vi "transformedStadisticColumnInformation.vi"(8 "error in":errorcluster, 11 "columnInformationReading":T2(array[cluster])) -> (0 "error out":errorcluster, 3 "columnInformationReadingTransformed":string[](array[string]))   [LabVIEW 2014]
uses:
  <vilib>/addons/database/Auxilliary.llb/DB Tools DataTypes.ctl
  <vilib>/addons/database/NI_Database_API.lvlib
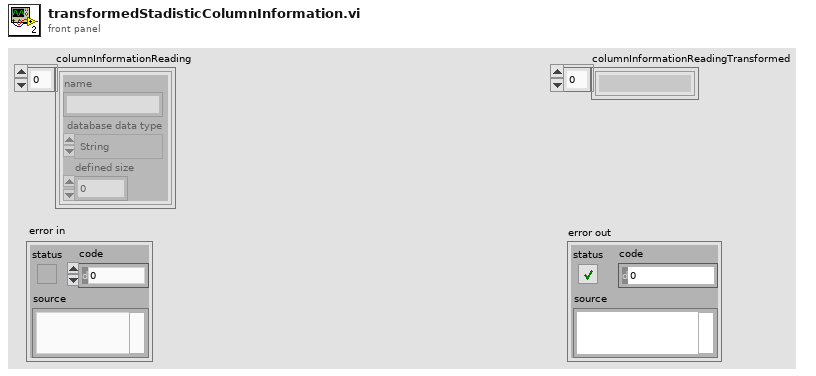
[diagram p1: front panel]
types:
  T1 = typedef "NI_Database_API.lvlib/DB Tools DataTypes.ctl" = enum16{"String", "Long (I32)", "Single (SGL)", "Double (DBL)", "Date/Time", "Binary"}
  T2 = cluster{"name":string, "database data type":T1, "defined size":i32}[]
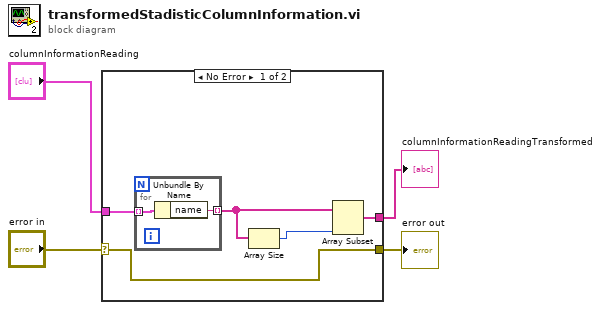
[diagram p0: block diagram]
diagram:
  n1 = case shown="No Error" "error in" {
    selector: "error in" -> [w6 w12]
    tunnel: "columnInformationReading" -> [w9 _]
    tunnel: [w8 _] -> w3
    tunnel: [w6 w12] -> w1
    frame No Error {
      n2 = for {
        tunnel: w9 -> [w10] mode=indexing
        tunnel: [w11] -> w7 mode=indexing
        n3 = Unbundle By Name(w10) -> ("name"=w11:string)
      }
      n4 = Array Size(array=w7) -> (size(s)=w5:i32)
      n5 = Array Subset(array=w7, length=w5) -> (w8:string[])  [unwired: 1 in]
    }
    frame Error {
    }
  }
  "columnInformationReadingTransformed" <- w3
  "error out" <- w1
